vi "InTake Global Data.vi"() -> ()   [LabVIEW 2013]
panel:
  in  "InTake Global Data In":T1
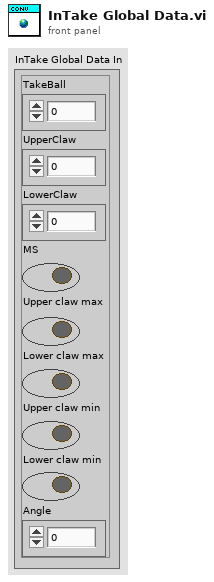
[diagram p1: front panel]
types:
  T1 = cluster{"TakeBall":dbl, "UpperClaw":dbl, "LowerClaw":dbl, "MS":bool, "Upper claw max":bool, "Lower claw max":bool, "Upper claw min":bool, "Lower claw min":bool, "Angle":dbl}
diagram:
